vi "Trim Log File.vi"(9 "Trim n entries":i32, 10 "Fault Log Contents":string, 11 "Fault Message":string) -> (2 "Trimmed Fault Log":string)   [LabVIEW 2014]
doc: "Removes the \"n\" oldest entries from the input string of XML-RPC Fault Messages"
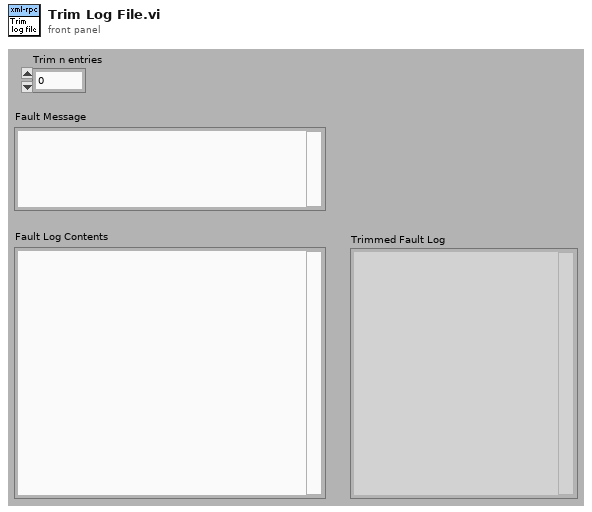
[diagram p1: front panel]
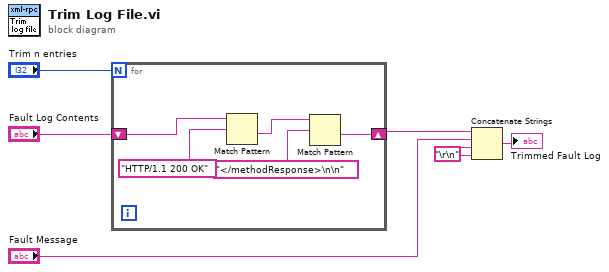
[diagram p0: block diagram]
diagram:
  w2 = "\r\n"
  n1 = for {
    N: "Trim n entries" -> [_]
    shift-right: [w7] -> w4
    shift-left: "Fault Log Contents" -> [w11]
    n2 = Match Pattern(string=w11, regular expression="HTTP/1.1 200 OK") -> (after substring=w9:string)  [unwired: 1 in, 3 out]
    n3 = Match Pattern(string=w9, regular expression="</methodResponse>\n\n") -> (after substring=w7:string)  [unwired: 1 in, 3 out]
  }
  n4 = Concatenate Strings(w4, "Fault Message", w2, w2) -> (→"Trimmed Fault Log":string)
